vi "Comments.Create Lockin REF Description.vi"(7 "error in (no error)":errorcluster, 10 "Control Experiment":refnum<class "Control Experiment.lvclass">) -> (0 "error out":errorcluster, 2 "REF Section":string, 3 "Control Experiment out":refnum<class "Control Experiment.lvclass">)   [LabVIEW 2019, in "Control Experiment.lvclass"]
uses:
  Control Experiment.lvclass
  Control Experiment.lvclass/Control Experiment.ctl
  <userlib>/LevyLab/Lockin-Multichannel/Instrument.Lockin/Instrument.Lockin.lvclass
  <userlib>/LevyLab/PLYM/YAML.lvclass
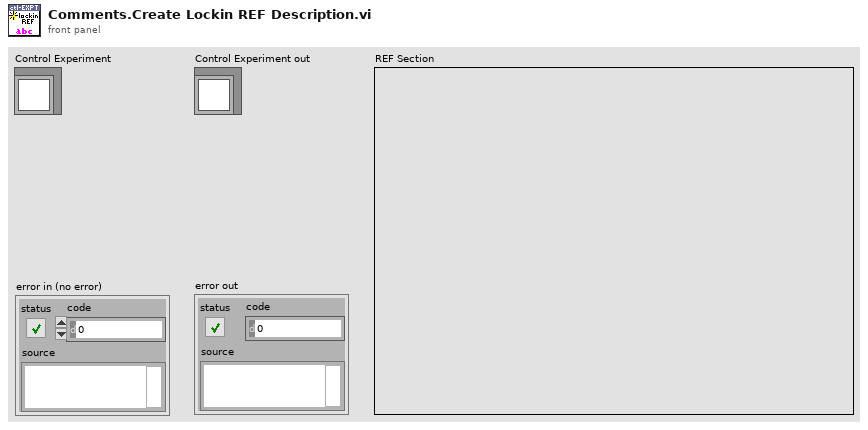
[diagram p1: front panel]
types:
  T1 = typedef "Lockin.DAQ.lvclass/REF-cluster.ctl" = T2[]
  T2 = typedef "Instrument.Lockin.UI.lvclass/REF Channel--Cluster.ctl" = cluster{"Enable?":bool, "Channel":i32, "Frequency":dbl, "Phase":dbl, "TC":dbl, "Roll-Off":i32}
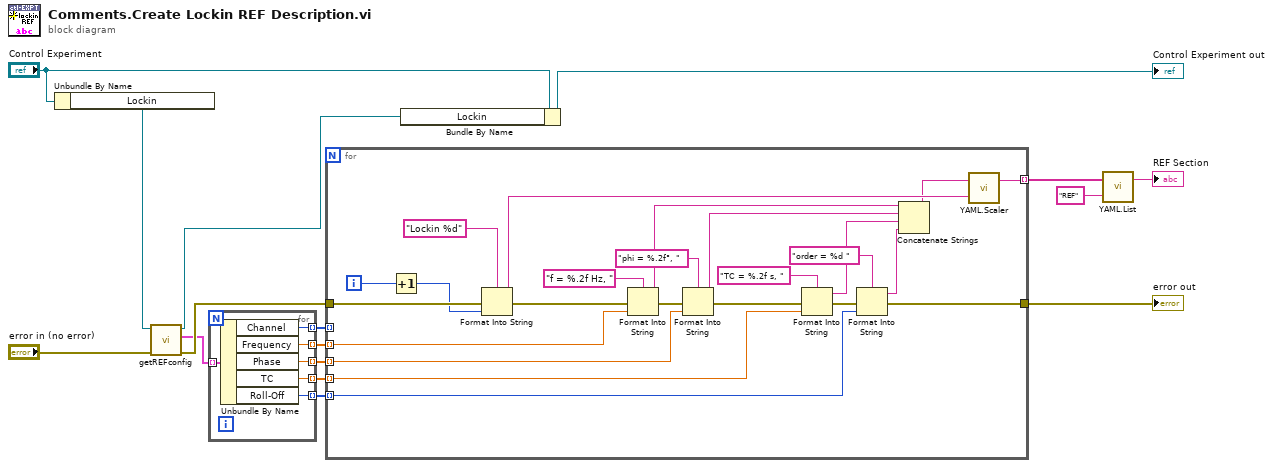
[diagram p0: block diagram]
diagram:
  n1 = Unbundle By Name("Control Experiment") -> ("Lockin"=w9:refnum<class "Instrument.Lockin.lvclass">)
  n2 = call <userlib>:"getREFconfig.vi"("error in (no error)"="error in (no error)", "Instrument.Lockin in"=w9) -> ("error out"=w5:errorcluster, "REFconfig"=w4:T1, "Instrument.Lockin out"=w1:refnum<class "Instrument.Lockin.lvclass">)  [unwired: 7 in]
  n3 = for {
    tunnel: [w22] -> w16 mode=indexing
    tunnel: [w21] -> w15 mode=indexing
    tunnel: w4 -> [w20] mode=indexing
    tunnel: [w19] -> w8 mode=indexing
    tunnel: [w18] -> w7 mode=indexing
    tunnel: [w17] -> w6 mode=indexing
    n4 = Unbundle By Name(w20) -> ("Channel"=w22:i32, "Frequency"=w21:dbl, "Phase"=w19:dbl, "TC"=w18:dbl, "Roll-Off"=w17:i32)
  }
  n5 = for {
    tunnel: w16 -> [_] mode=indexing
    tunnel: w15 -> [w32] mode=indexing
    tunnel: w5 -> [w46]
    tunnel: [w27] -> w14
    tunnel: [w35] -> w10 mode=indexing
    tunnel: w8 -> [w33] mode=indexing
    tunnel: w7 -> [w26] mode=indexing
    tunnel: w6 -> [w25] mode=indexing
    i -> [w44]
    n6 = Increment(x=w44) -> (x+1=w34:i32)
    n7 = Format Into String(format string="Lockin %d", error in=w46, w34) -> (resulting string=w37:string, error out=w39:errorcluster)  [unwired: 1 in]
    n8 = Format Into String(format string="f = %.2f Hz, ", error in=w39, w32) -> (resulting string=w41:string, error out=w45:errorcluster)  [unwired: 1 in]
    n9 = Format Into String(format string="phi = %.2f°, ", error in=w45, w33) -> (resulting string=w40:string, error out=w28:errorcluster)  [unwired: 1 in]
    n10 = Format Into String(format string="TC = %.2f s, ", error in=w28, w26) -> (resulting string=w23:string, error out=w29:errorcluster)  [unwired: 1 in]
    n11 = Format Into String(format string="order = %d ", error in=w29, w25) -> (resulting string=w24:string, error out=w27:errorcluster)  [unwired: 1 in]
    n12 = Concatenate Strings(w41, w40, w23, w24) -> (w36:string)
    n13 = call <userlib>:"YAML.Scaler.vi"("Key"=w37, "Scaler"=w36) -> ("Output"=w35:string)  [unwired: 1 in]
  }
  "error out" <- w14
  n14 = Bundle By Name(cluster="Control Experiment", "Lockin"=w1) -> (→"Control Experiment out":refnum<class "Control Experiment.lvclass">)
  n15 = call <userlib>:"YAML.List.vi"("Key"="REF" ("string"), "lines"=w10) -> ("Output"=→"REF Section":string)  [unwired: 1 in]
